vi "Header Footer Create Cell.vi"(0 "Change format?":bool, 1 "Header or Footer":T13, 2 "FixedHeight (points)":sgl, 3 "Padding (points)":sgl, 7 "Header Footer Cluster with references IN":T1={"Start page"=1, "Type"=enum."Select", "Start with #"=1, "Alignment"=enum."Center", "Vertical Alignement"=enum."MIDDLE", "Page #"={"Text 1"="", "Text 2"="", "Text 3"=""}, "Text"=refnum, "Scaled Img"=refnum, "PdfPCell"=refnum, "PdfPTable"=refnum, "Font Cluster"={"Name"="", "Size"=-1.0, "Color"=0, "Style"={"Bold"=FALSE, "Italic"=FALSE, "Underline"=FALSE, "Strikeout"=FALSE}, "Type"={"Type&direction"=enum."Select", "Embedded"=FALSE, "Encoding"=""}}, "Font "=refnum, "Img (%)"=100.0, "Line"={"Line"=enum."Horizontal line", "Thickness (points)"=0.75, "Colour"=7171459}, "Line spacing"=enum."Select"}, 11 "error in (no error)":errorcluster) -> (4 "PdfP Cell":refnum<k24>, 8 "Header Footer Cluster with references OUT":T1={"Start page"=1, "Type"=enum."Select", "Start with #"=1, "Alignment"=enum."Center", "Vertical Alignement"=enum."MIDDLE", "Page #"={"Text 1"="", "Text 2"="", "Text 3"=""}, "Text"=refnum, "Scaled Img"=refnum, "PdfPCell"=refnum, "PdfPTable"=refnum, "Font Cluster"={"Name"="", "Size"=-1.0, "Color"=0, "Style"={"Bold"=FALSE, "Italic"=FALSE, "Underline"=FALSE, "Strikeout"=FALSE}, "Type"={"Type&direction"=enum."Select", "Embedded"=FALSE, "Encoding"=""}}, "Font "=refnum, "Img (%)"=100.0, "Line"={"Line"=enum."Horizontal line", "Thickness (points)"=0.75, "Colour"=7171459}, "Line spacing"=enum."Select"}, 15 "error out":errorcluster)   [LabVIEW 2019, in "Exaprom PDF.lvlib"]
doc: "Version 1.0\nDeveloped by Jean-Marc Simard\nCopyright © 2010, Exaprom Inc.\nAll rights reserved.\nLicense: BSD\n\nWith iTextSharp 4.1.6 (http://itextsharp.sourceforge.net)\nunder Mozilla Public License Version 1.1\n(http://www.mozilla.org/MPL/MPL-1.1.html)"
uses:
  C:/work/niobrara_lv/labview pdf writer fixing/DLL/itextsharp.dll
  DLL/itextsharp.dll
  Controls/Header, Footer and Watermark Controls/Header Footer Cluster with references.ctl
  Controls/Header, Footer and Watermark Controls/Header Footer Type.ctl
  Controls/Header, Footer and Watermark Controls/Header footer horiz alignment.ctl
  Controls/Table Controls/Cell Vertical alignment.ctl
  Controls/Header, Footer and Watermark Controls/Page number.ctl
  Controls/Font Controls/Font complete cluster horizontal.ctl
  Controls/Font Controls/Font size.ctl
  Controls/Font Controls/Font color.ctl
  Controls/Font Controls/Type and encoding.ctl
  Controls/Text Controls/Unicode/Type and run direction.ctl
  Controls/Header, Footer and Watermark Controls/Header Footer Line.ctl
  Controls/Text Controls/Line spacing.ctl
  Controls/Header, Footer and Watermark Controls/Header or Footer.ctl
  Exaprom PDF.lvlib
panel:
  # "X"
  # "Y"
  # "X"
  # "Y"
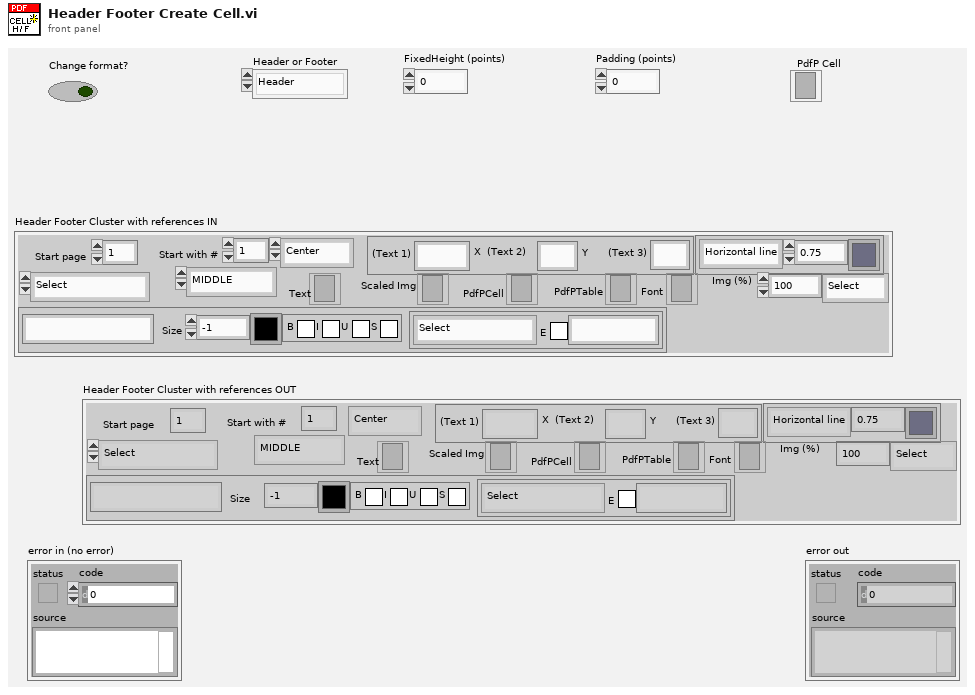
[diagram p1: front panel]
types:
  T1 = typedef "Exaprom PDF.lvlib/Header Footer Cluster with references.ctl" = cluster{"Start page":i32, "Type":T2, "Start with #":i32, "Alignment":T3, "Vertical Alignement":T4, "Page #":T5, "Text":refnum<k24>, "Scaled Img":refnum<k24>, "PdfPCell":refnum<k24>, "PdfPTable":refnum<k24>, "Font Cluster":T6, "Font ":refnum<k24>, "Img (%)":sgl, "Line":cluster{"Line":T11, "Thickness (points)":sgl, "Colour":T8}, "Line spacing":T12}
  T2 = typedef "Exaprom PDF.lvlib/Header Footer Type.ctl" = enum16{"Select", "Text", "Text + hyperlink", "Page number", "Image", "Image + hyperlink"}
  T3 = typedef "Exaprom PDF.lvlib/Header footer horiz alignment.ctl" = enum16{"Left", "Center", "Right"}
  T4 = typedef "Exaprom PDF.lvlib/Cell Vertical alignment.ctl" = enum16{"TOP", "MIDDLE", "BOTTOM"}
  T5 = typedef "Exaprom PDF.lvlib/Page number.ctl" = cluster{"Text 1":string, "Text 2":string, "Text 3":string}
  T6 = typedef "Exaprom PDF.lvlib/Font complete cluster horizontal.ctl" = cluster{"Name":string, "Size":T7, "Color":T8, "Style":cluster{"Bold":bool, "Italic":bool, "Underline":bool, "Strikeout":bool}, "Type":T9}
  T7 = typedef "Exaprom PDF.lvlib/Font size.ctl" = sgl
  T8 = typedef "Exaprom PDF.lvlib/Font color.ctl" = u32
  T9 = typedef "Exaprom PDF.lvlib/Type and encoding.ctl" = cluster{"Type&direction":T10, "Embedded":bool, "Encoding":string}
  T10 = typedef "Exaprom PDF.lvlib/Type and run direction.ctl" = enum16{"Select", "ASCII", "UTF-16", "UTF-16 (default)", "UTF-16 (LTR)", "UTF-16 (RTL)"}
  T11 = typedef "Exaprom PDF.lvlib/Header Footer Line.ctl" = enum16{"No line", "Horizontal line"}
  T12 = typedef "Exaprom PDF.lvlib/Line spacing.ctl" = enum16{"Select", "1.0", "1.5", "2.0"}
  T13 = typedef "Exaprom PDF.lvlib/Header or Footer.ctl" = enum16{"Header", "Footer"}
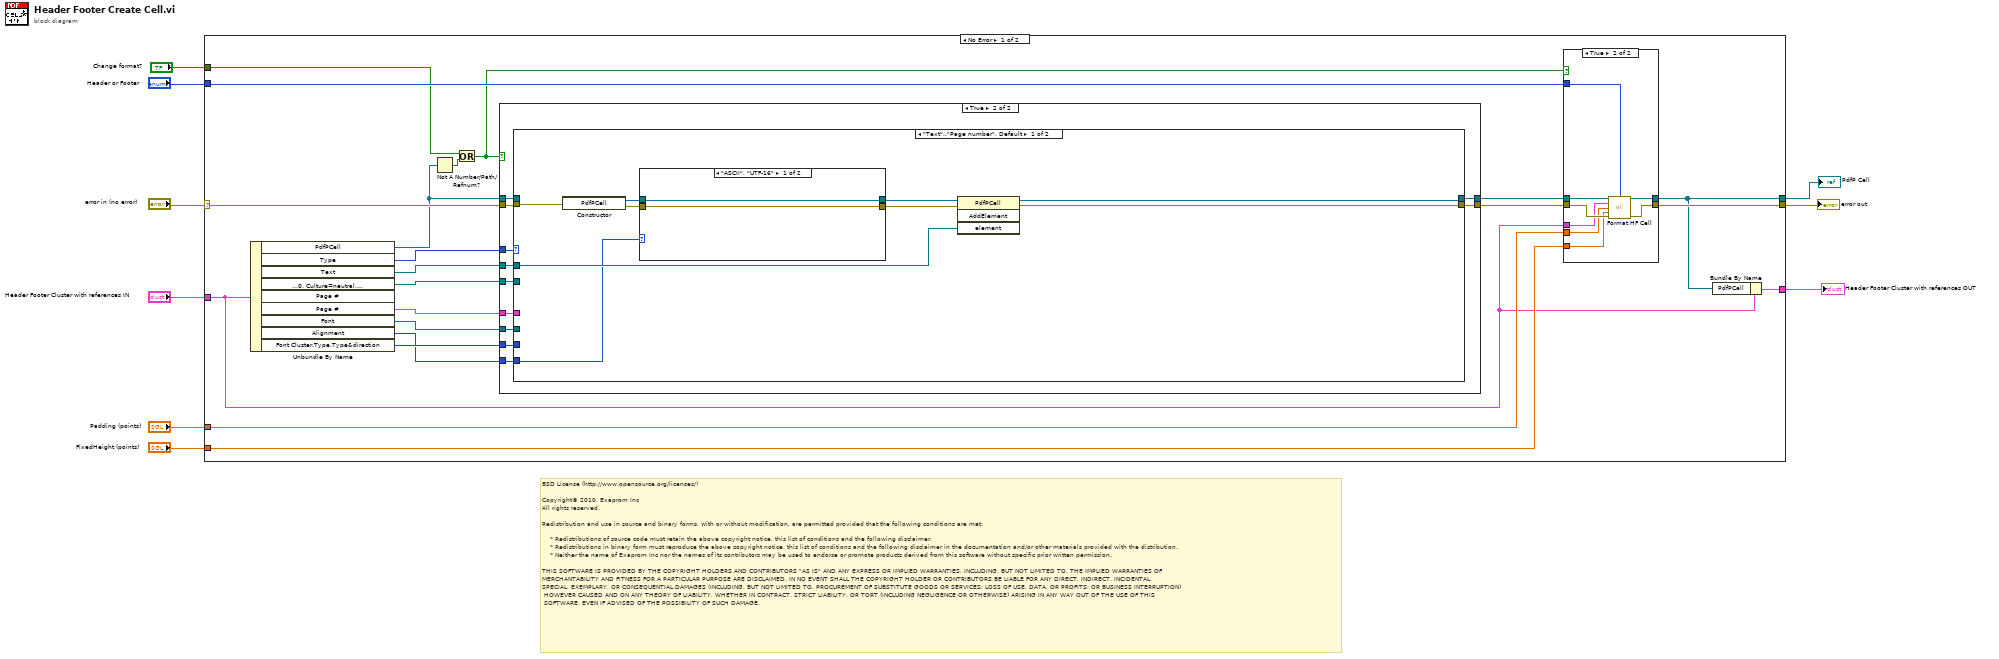
[diagram p0: block diagram]
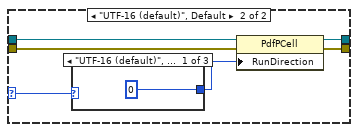
[diagram p3: hidden frame]
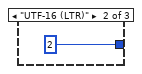
[diagram p4: hidden frame]
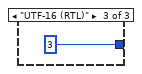
[diagram p5: hidden frame]
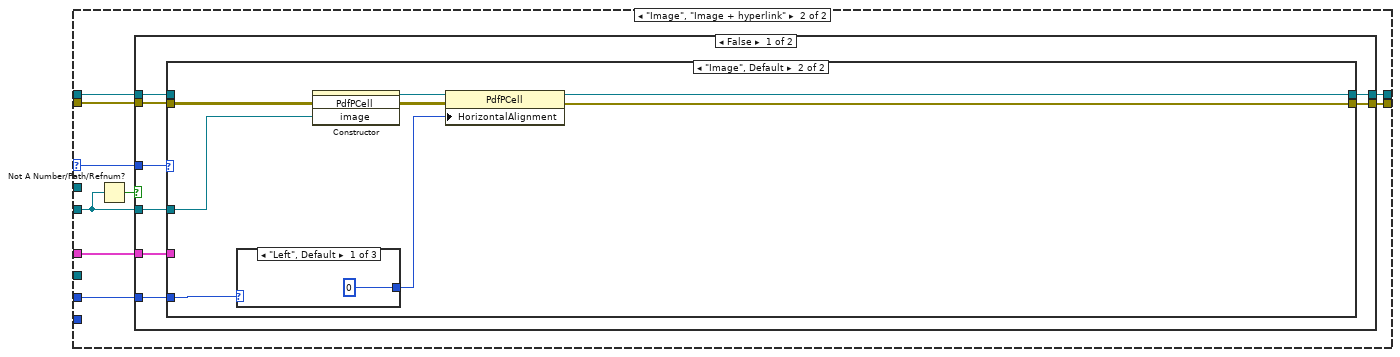
[diagram p6: hidden frame]
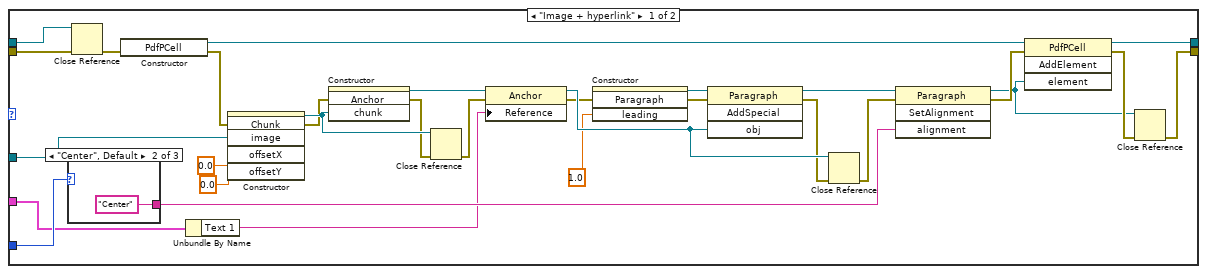
[diagram p7: hidden frame]
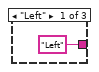
[diagram p8: hidden frame]
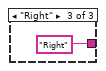
[diagram p9: hidden frame]
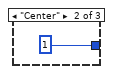
[diagram p10: hidden frame]
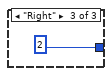
[diagram p11: hidden frame]
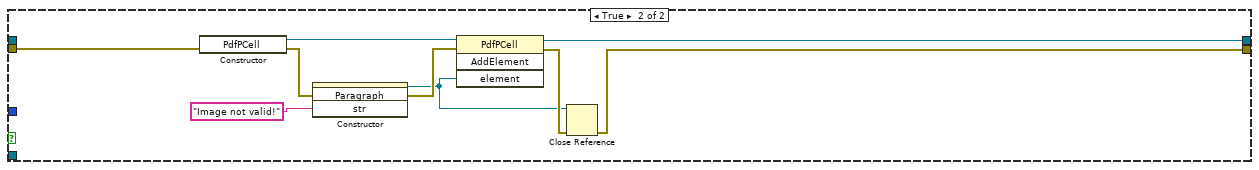
[diagram p12: hidden frame]
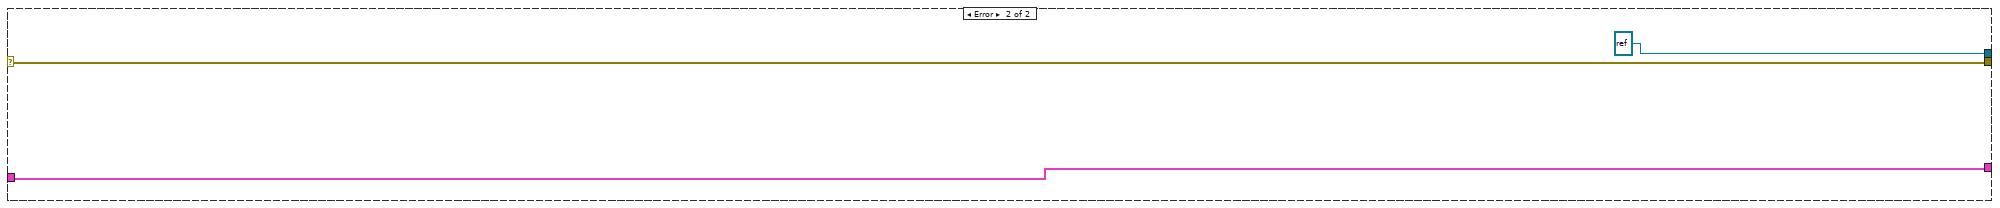
[diagram p14: hidden frame]
diagram:
  # "BSD License (http://www.opensource.org/licenses/)\n\nCopyright© 2010, Exaprom Inc\nAll rights reserved.\n\nRedistribution and use in source and binary forms, with or without modification, are permitted provided that the following conditions are met:\n\n    * Redistributions of source code must retain the above copyright notice, this list of conditions and the following disclaimer.\n    * Redistributions in binary form must reproduce the above copyright notice, this list of conditions and the following disclaimer in the documentation and/or other materials provided with the distribution.\n    * Neither the name of Exaprom Inc nor the names of its contributors may be used to endorse or promote products derived from this software without specific prior written permission.\n\nTHIS SOFTWARE IS PROVIDED BY THE COPYRIGHT HOLDERS AND CONTRIBUTORS \"AS IS\" AND ANY EXPRESS OR IMPLIED WARRANTIES, INCLUDING, BUT NOT LIMITED TO, THE IMPLIED WARRANTIES OF \nMERCHANTABILITY AND FITNESS FOR A PARTICULAR PURPOSE ARE DISCLAIMED. IN NO EVENT SHALL THE COPYRIGHT HOLDER OR CONTRIBUTORS BE LIABLE FOR ANY DIRECT, INDIRECT, INCIDENTAL,\nSPECIAL, EXEMPLARY, OR CONSEQUENTIAL DAMAGES (INCLUDING, BUT NOT LIMITED TO, PROCUREMENT OF SUBSTITUTE GOODS OR SERVICES; LOSS OF USE, DATA, OR PROFITS; OR BUSINESS INTERRUPTION)\n HOWEVER CAUSED AND ON ANY THEORY OF LIABILITY, WHETHER IN CONTRACT, STRICT LIABILITY, OR TORT (INCLUDING NEGLIGENCE OR OTHERWISE) ARISING IN ANY WAY OUT OF THE USE OF THIS\n SOFTWARE, EVEN IF ADVISED OF THE POSSIBILITY OF SUCH DAMAGE."
  n1 = case shown="No Error" "error in (no error)" {
    selector: "error in (no error)" -> [w30 w146]
    tunnel: [w13 refnum<k24> refnum ("new reference")] -> w9
    tunnel: [w23 w146] -> w8
    tunnel: "Header Footer Cluster with references IN" -> [w14 w144]
    tunnel: "Padding (points)" -> [w22 _]
    tunnel: "FixedHeight (points)" -> [w21 _]
    tunnel: "Header or Footer" -> [w20 _]
    tunnel: "Change format?" -> [w12 _]
    tunnel: [w15 w144] -> w1
    frame No Error {
      n2 = Unbundle By Name(w14) -> ("PdfPCell"=w18:refnum<k24>, "Type"=w17:T2, "Text"=w28:refnum<k24>, "Scaled Img"=w29:refnum<k24>, "Page #"=w19:T5, "Font"=w27:refnum<k24>, "Alignment"=w26:T3, "Font Cluster.Type.Type&direction"=w10:T10)  [unwired: 1 out]
      n3 = Not A Number/Path/Refnum?(number/path/refnum=w18) -> (NaN/Path/Refnum?=w16:bool)
      n4 = Or(x=w12, y=w16) -> (x .or. y?=w11:bool)
      n5 = case shown="True" w11 {
        tunnel: [w32 w43] -> w25
        tunnel: [w31 w42] -> w24
        tunnel: w17 -> [_ w41]
        tunnel: w30 -> [w31 w40]
        tunnel: w29 -> [_ w39]
        tunnel: w19 -> [_ w38]
        tunnel: w28 -> [_ w37]
        tunnel: w27 -> [_ w36]
        tunnel: w26 -> [_ w35]
        tunnel: w18 -> [w32 w34]
        tunnel: w10 -> [_ w33]
        frame False {
        }
        frame True {
          n6 = case shown="\"Text\"..\"Page number\", Default" w41 {
            selector: w41 -> [_ w69]
            tunnel: [w50 w72] -> w43
            tunnel: w36 -> [_ _]
            tunnel: w35 -> [_ w70]
            tunnel: [w49 w71] -> w42
            tunnel: w40 -> [w51 w68]
            tunnel: w39 -> [_ w66]
            tunnel: w38 -> [_ w67]
            tunnel: w37 -> [w52 _]
            tunnel: w34 -> [_ w64]
            tunnel: w33 -> [w44 _]
            frame "Text".."Page number", Default {
              n7 = constructor class="PdfPCell"(error in=w51) -> (reference out=w48:refnum<k24>, error out=w45:errorcluster)  [unwired: 2 in, 1 out]
              n8 = case shown="\"ASCII\", \"UTF-16\"" w44 {
                selector: w44 -> [_ w56]
                tunnel: w48 -> [w54 w60]
                tunnel: [w54 w59] -> w47
                tunnel: [w53 w58] -> w46
                tunnel: w45 -> [w53 w57]
                frame "ASCII", "UTF-16" {
                }
                frame "UTF-16 (default)", Default {
                  n9 = case shown="\"UTF-16 (default)\", Default" w56 {
                    tunnel: [0 ("RunDirection") 2 ("RunDirection") 3 ("RunDirection")] -> w55
                    frame "UTF-16 (default)", Default {
                    }
                    frame "UTF-16 (LTR)" {
                    }
                    frame "UTF-16 (RTL)" {
                    }
                  }
                  n10 = property class="PdfPCell"(reference=w60, error in=w57, "RunDirection"=w55) -> (reference out=w59:refnum<k24>, error out=w58:errorcluster)
                }
              }
              n11 = invoke class="PdfPCell" method="AddElement"(reference=w47, error in=w46, "element"=w52) -> (reference out=w50:refnum<k24>, error out=w49:errorcluster)  [unwired: 1 in, 2 out]
            }
            frame "Image", "Image + hyperlink" {
              n12 = Not A Number/Path/Refnum?(number/path/refnum=w66) -> (NaN/Path/Refnum?=w65:bool)
              n13 = case shown="False" w65 {
                tunnel: [w78 w126] -> w71
                tunnel: [w79 w130] -> w72
                tunnel: w70 -> [w80 _]
                tunnel: w69 -> [w77 _]
                tunnel: w68 -> [w75 w125]
                tunnel: w66 -> [w76 _]
                tunnel: w67 -> [w74 _]
                tunnel: w64 -> [w73 _]
                frame False {
                  n14 = case shown="\"Image\", Default" w77 {
                    tunnel: w80 -> [w88 w121]
                    tunnel: [w90 w118] -> w79
                    tunnel: w75 -> [w89 w116]
                    tunnel: [w87 w114] -> w78
                    tunnel: w74 -> [w86 _]
                    tunnel: w76 -> [w84 w115]
                    tunnel: w73 -> [w81 _]
                    frame "Image + hyperlink" {
                      n15 = case shown="\"Center\", Default" w88 {
                        tunnel: ["Left" "Center" "Right"] -> w107
                        frame "Left" {
                        }
                        frame "Center", Default {
                        }
                        frame "Right" {
                        }
                      }
                      n16 = Close Reference(reference=w81, error in (no error)=w89) -> (error out=w82:errorcluster)
                      n17 = constructor class="PdfPCell"(error in=w82) -> (reference out=w106:refnum<k24>, error out=w95:errorcluster)  [unwired: 2 in, 1 out]
                      n18 = Unbundle By Name(w86) -> ("Text 1"=w83:string)
                      n19 = constructor class="Chunk"(error in=w95, "image"=w84, "offsetX"=sgl 0.0, "offsetY"=sgl 0.0) -> (reference out=w110:refnum<k24>, error out=w91:errorcluster)  [unwired: 2 in, 4 out]
                      n20 = constructor class="Anchor"(error in=w91, "chunk"=w110) -> (reference out=w94:refnum<k24>, error out=w108:errorcluster)  [unwired: 2 in, 2 out]
                      n21 = Close Reference(reference=w110, error in (no error)=w108) -> (error out=w109:errorcluster)
                      n22 = property class="Anchor"(reference=w94, error in=w109, "Reference"=w83) -> (reference out=w105:refnum<k24>, error out=w104:errorcluster)
                      n23 = constructor class="Paragraph"(error in=w104, "leading"=sgl 1.0) -> (reference out=w100:refnum<k24>, error out=w101:errorcluster)  [unwired: 2 in, 2 out]
                      n24 = invoke class="Paragraph" method="AddSpecial"(reference=w100, error in=w101, "obj"=w105) -> (reference out=w102:refnum<k24>, error out=w99:errorcluster)  [unwired: 1 in, 2 out]
                      n25 = Close Reference(reference=w105, error in (no error)=w99) -> (error out=w98:errorcluster)
                      n26 = invoke class="Paragraph" method="SetAlignment"(reference=w102, error in=w98, "alignment"=w107) -> (reference out=w96:refnum<k24>, error out=w103:errorcluster)  [unwired: 1 in, 2 out]
                      n27 = invoke class="PdfPCell" method="AddElement"(reference=w106, error in=w103, "element"=w96) -> (reference out=w90:refnum<k24>, error out=w97:errorcluster)  [unwired: 1 in, 2 out]
                      n28 = Close Reference(reference=w96, error in (no error)=w97) -> (error out=w87:errorcluster)
                    }
                    frame "Image", Default {
                      n29 = case shown="\"Left\", Default" w121 {
                        tunnel: [0 1 2] -> w117
                        frame "Left", Default {
                        }
                        frame "Center" {
                        }
                        frame "Right" {
                        }
                      }
                      n30 = constructor class="PdfPCell"(error in=w116, "image"=w115) -> (reference out=w120:refnum<k24>, error out=w119:errorcluster)  [unwired: 2 in, 2 out]
                      n31 = property class="PdfPCell"(reference=w120, error in=w119, "HorizontalAlignment"=w117) -> (reference out=w118:refnum<k24>, error out=w114:errorcluster)
                    }
                  }
                }
                frame True {
                  n32 = constructor class="PdfPCell"(error in=w125) -> (reference out=w131:refnum<k24>, error out=w133:errorcluster)  [unwired: 2 in, 1 out]
                  n33 = constructor class="Paragraph"(error in=w133, "str"="Image not valid!") -> (reference out=w127:refnum<k24>, error out=w132:errorcluster)  [unwired: 2 in, 2 out]
                  n34 = invoke class="PdfPCell" method="AddElement"(reference=w131, error in=w132, "element"=w127) -> (reference out=w130:refnum<k24>, error out=w128:errorcluster)  [unwired: 1 in, 2 out]
                  n35 = Close Reference(reference=w127, error in (no error)=w128) -> (error out=w126:errorcluster)
                }
              }
            }
          }
        }
      }
      n36 = case shown="True" w11 {
        tunnel: w25 -> [w135 w143]
        tunnel: w24 -> [w134 w141]
        tunnel: [w135 w142] -> w13
        tunnel: [w134 w140] -> w23
        tunnel: w14 -> [_ w139]
        tunnel: w22 -> [_ w138]
        tunnel: w21 -> [_ w137]
        tunnel: w20 -> [_ w136]
        frame False {
        }
        frame True {
          n37 = call "Format HF Cell.vi"("PdfP Cell"=w143, "Header or Footer"=w136, "Header Footer Cluster with references"=w139, "Padding (points)"=w138, "FixedHeight (points)"=w137, "error in (no error)"=w141) -> ("PdfP Cell duplicate"=w142:refnum<k24>, "error out"=w140:errorcluster)  [unwired: 8 out]
        }
      }
      n38 = Bundle By Name(cluster=w14, "PdfPCell"=w13) -> (w15:T1)
    }
    frame Error {
    }
  }
  "PdfP Cell" <- w9
  "error out" <- w8
  "Header Footer Cluster with references OUT" <- w1
